vi "PDA_Temperature_Readout.vi"(0 "stop":bool, 1 "msec to wait":u32=1000, 3 "error in":errorcluster, 4 "Init InGaAs":bool) -> (5 "PDA Temperature":dbl(graph), 7 "error out":errorcluster)   [LabVIEW 2019]
uses:
  Globals and TypeDefs/Type Definitions.llb/3 way Status.ctl
  Globals and TypeDefs/gStatus.vi
panel:
  in  "CCD ADC and Gain":dbl(ring) items=["16 bits Gain 1", "16 bits Gain 2"]
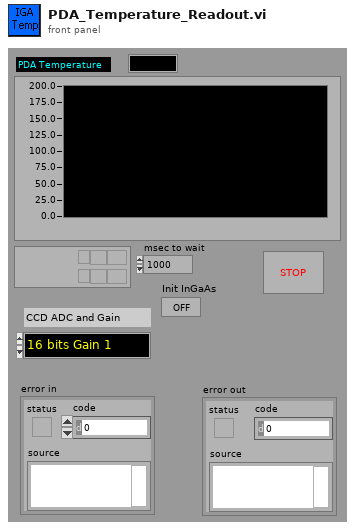
[diagram p1: front panel]
types:
  T1 = enum16{"CCD Temperature Z345", "CCD Temperature Z308", "CCD Gain"}
  T2 = typedef "3 way Status.ctl" = u8
  T3 = cluster{"Comm Interface":u16, "BUS":i16, "Address":i16, "Com Port":i32}
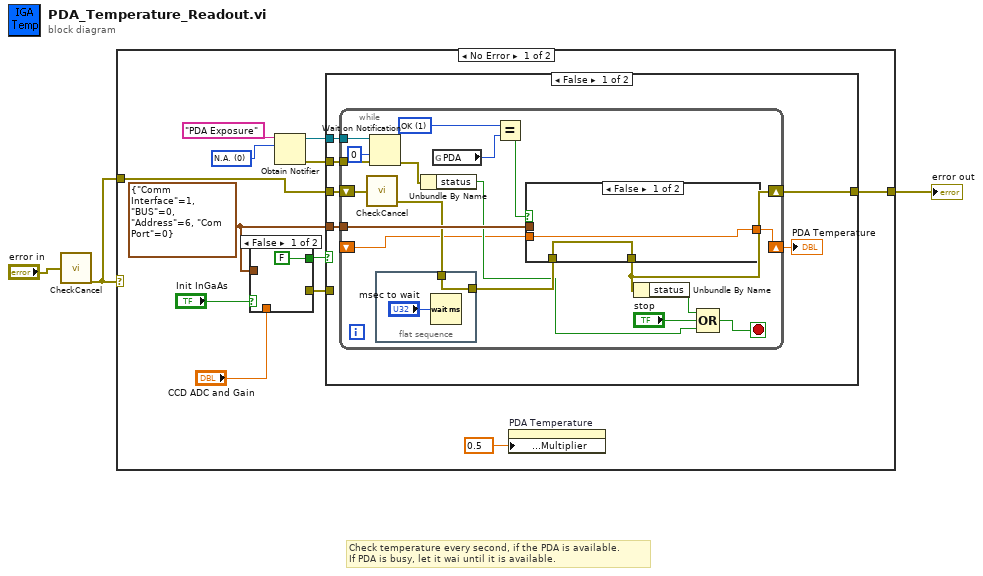
[diagram p0: block diagram]
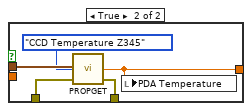
[diagram p2: hidden frame]
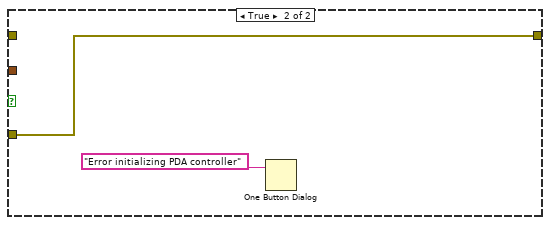
[diagram p3: hidden frame]
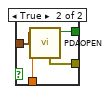
[diagram p4: hidden frame]
diagram:
  # "Check temperature every second, if the PDA is available. \nIf PDA is busy, let it wai until it is available."
  n1 = call "CheckCancel.vi"("error in (no error)"="error in") -> ("error out"=w2:errorcluster)  [unwired: 1 in, 1 out]
  n2 = case shown="No Error" w2 {
    tunnel: w2 -> [w11 w56]
    tunnel: [w10 w56] -> w1
    frame No Error {
      w7 = T2 0 items=["N.A.", "OK", "Busy", "Done"] ("Saving")
      w15 = T3 {"Comm Interface"=1, "BUS"=0, "Address"=6, "Com Port"=0} ("Comm Params")
      n3 = case shown="False" "Init InGaAs" {
        tunnel: [FALSE ("Boot Error") w55] -> w14
        tunnel: w15 -> [_ w54]
        tunnel: "CCD ADC and Gain" -> [_ w53]
        tunnel: [_ w52] -> w9
        frame False {
        }
        frame True {
          n4 = call "PDAOPEN.VI"("CCD ADC and Gain"=w53, "Comm Params"=w54) -> ("error out"=w52:errorcluster, "Boot Error"=w55:bool)  [unwired: 1 in, 4 out]
        }
      }
      n5 = Obtain Notifier(name (unnamed)="PDA Exposure", notification data type=w7) -> (notifier out=w5:refnum<notifier>, error out=w4:errorcluster)  [unwired: 2 in, 1 out]
      n6 = case shown="False" w14 {
        tunnel: w15 -> [w21 _]
        tunnel: w11 -> [w20 _]
        tunnel: [w19 w49] -> w10
        tunnel: w9 -> [_ w49]
        tunnel: w5 -> [w18 _]
        tunnel: w4 -> [w17 _]
        frame False {
          n7 = while {
            tunnel: w21 -> [w39]
            shift-right: [w34] -> w19
            shift-left: w20 -> [w36]
            tunnel: w18 -> [w32]
            tunnel: w17 -> [w31]
            shift-right: [w23] -> w16
            shift-left: _ -> [w22]
            stop <- w37 stop-if-true
            w28 = T2 1 items=["N.A.", "OK", "Busy", "Done"] ("x")
            n8 = call "CheckCancel.vi"("error in (no error)"=w36) -> ("error out"=w33:errorcluster)  [unwired: 1 in, 1 out]
            n9 = Wait on Notification(notifier=w32, timeout in ms (-1)=0, error in (no error)=w31) -> (error out=w29:errorcluster)  [unwired: 1 in, 3 out]
            n10 = flat-sequence {
              tunnel: w33 -> [w48]
              tunnel: [w48] -> w26
              frame #0 {
                n11 = Wait (ms)(milliseconds to wait="msec to wait") -> ()  [unwired: 1 out]
              }
            }
            n12 = Unbundle By Name(w29) -> ("status"=w25:bool)
            n13 = global read "gStatus.vi" "PDA"() -> (w24:T2)
            n14 = Equal?(x=w28, y=w24) -> (x = y?=w27:bool)
            n15 = case shown="False" w27 {
              tunnel: w39 -> [_ w46]
              tunnel: [w41 w44] -> w34
              tunnel: w26 -> [w41 w43]
              tunnel: [w40 w42] -> w23
              tunnel: w22 -> [w40 _]
              frame False {
              }
              frame True {
                n16 = call "PROPGET.VI"("error in"=w43, "CCD Prop ID"=T1."CCD Temperature Z345", "Comm Params"=w46) -> ("error out"=w44:errorcluster, "Output Param"=w42:dbl)  [unwired: 1 out]
                n17 = local write "PDA Temperature"(w42) -> ()
              }
            }
            n18 = Unbundle By Name(w34) -> ("status"=w35:bool)
            n19 = Compound Arithmetic op=OR(w35, "stop", w25) -> (w37:bool)
          }
          "PDA Temperature" <- w16
        }
        frame True {
          n20 = One Button Dialog(message="Error initializing PDA controller") -> ()  [unwired: 1 in, 1 out]
        }
      }
      n21 = property on="PDA Temperature" class="WFChart (strict)"("X Scale.Offset and Multiplier:Multiplier"=sgl 0.5 ("y")) -> ()  [unwired: 2 in, 2 out]
    }
    frame Error {
    }
  }
  "error out" <- w1
